vi "LVClass_ModalCoef Load From File.vi"(0 "ModalCoef in":refnum<class "ModalCoef.lvclass">, 5 "coefs_file_path":path, 11 "error in (no error)":errorcluster) -> (4 "ModalCoef out":refnum<class "ModalCoef.lvclass">, 8 "Comments":string, 15 "error out":errorcluster)   [LabVIEW 2020, in "ModalCoef.lvclass"]
doc: "ModalCoef constructor.\n\n--------------------------------------------------------------------------------\n\n<B>ModalCoefIn </B> : Constant Pointer to ModalCoef object.\n<B>ModalCoefOut </B> : Constant Pointer to ModalCoef object.\n<B>TypePhase </B> : TypePhase Phase mode reconstruction.\n<B>ErrorIn </B> : Error\n<B>ErrorOut </B> : Error\n\n--------------------------------------------------------------------------------"
uses:
  ModalCoef.lvclass
  ModalCoef.lvclass/ModalCoef.ctl
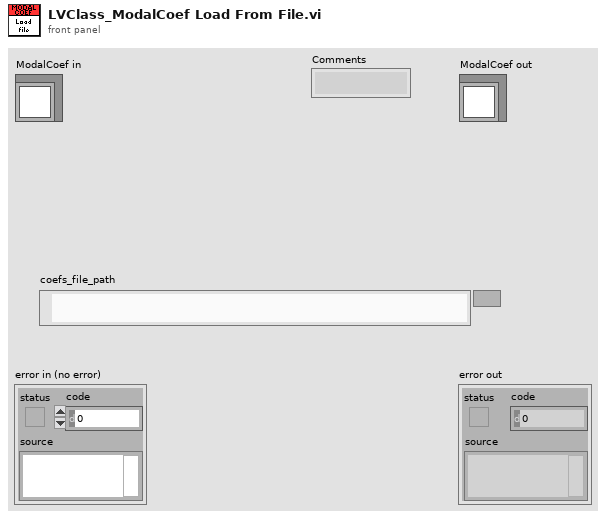
[diagram p1: front panel]
types:
  T1 = typedef "ClassID.ctl" = i64
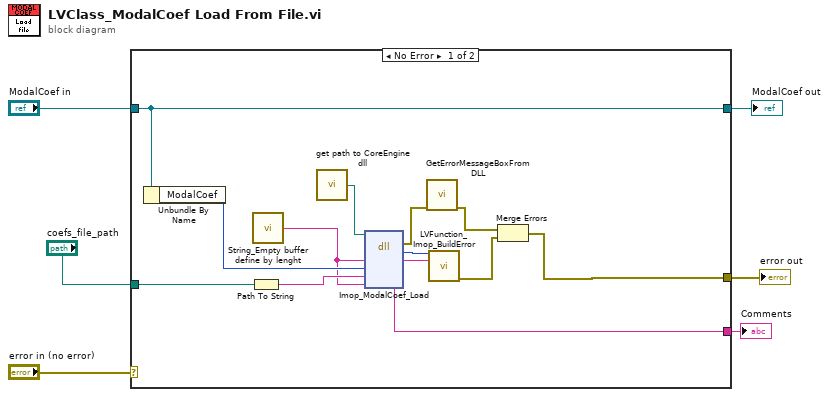
[diagram p0: block diagram]
diagram:
  n1 = case shown="No Error" "error in (no error)" {
    selector: "error in (no error)" -> [_ w21]
    tunnel: [w13 w21] -> w5
    tunnel: [w9 w20] -> w3
    tunnel: "ModalCoef in" -> [w9 w20]
    tunnel: "coefs_file_path" -> [w12 _]
    tunnel: [w7 _] -> w1
    frame No Error {
      n2 = Unbundle By Name(w9) -> ("ModalCoef"=w10:T1)
      n3 = Path To String(path=w12) -> (string=w11:string)
      n4 = call "String_Empty buffer define by lenght.vi"() -> ("Empty buffer"=w8:string)  [unwired: 1 in]
      n5 = call "get path to CoreEngine dll.vi"() -> ("path to wavekit library"=w17:path)  [unwired: 14 in, 1 out]
      n6 = dll-call lib="D:/soft/HASO_v3/SVN_trunk/ImOpCoreEngine4_LV2011/DLLs/c_interface_vc100.dll" fn="Imop_ModalCoef_Load"(path in=w17, "message"=w8, "ModalCoef"=w10, "coefs_file_path"=w11, "Comments"=w8) -> (error out=w16:errorcluster, "return type"=w18:i32, "message"=w19:string, "Comments"=w7:string)  [unwired: 4 in, 1 out]
      n7 = call "GetErrorMessageBoxFromDLL.vi"("error IN"=w16) -> ("error OUT"=w15:errorcluster)  [unwired: 10 in]
      n8 = call "LVFunction_Imop_BuildError.vi"("code"=w18, "String to Prepend to source (\"\")"=w19) -> ("error out"=w14:errorcluster)  [unwired: 13 in]
      n9 = Merge Errors(w15, w14) -> (w13:errorcluster)
    }
    frame Error {
    }
  }
  "error out" <- w5
  "ModalCoef out" <- w3
  "Comments" <- w1
